vi "Signal Amplitude Scaling.vi"(9 "Scaling Factor":dbl, 11 "Input":cdb[](array[numeric])) -> (3 "Output":cdb[](array[numeric]))   [LabVIEW 2022 SP3]
doc: "Signal scaling to prevent Peak-to-Average power Ratio (PAPR)"
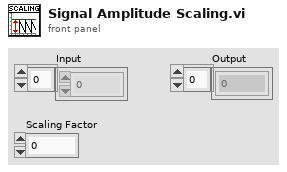
[diagram p1: front panel]
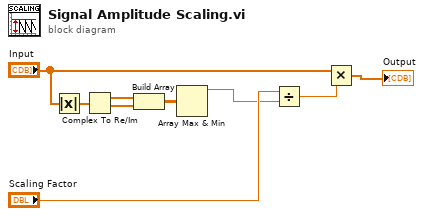
[diagram p0: block diagram]
diagram:
  n1 = Absolute Value(x="Input") -> (abs(x)=w9:dbl[])
  n2 = Complex To Re/Im(x + iy=w9) -> (x=w7:dbl[], y=w8:dbl[])
  n3 = Build Array(w7, w8) -> (w6:dbl[][])
  n4 = Array Max & Min(array=w6) -> (max value=w4:dbl)  [unwired: 3 out]
  n5 = Divide(x="Scaling Factor", y=w4) -> (x/y=w3:dbl)
  n6 = Multiply(x="Input", y=w3) -> (x*y=→"Output":cdb[])
